vi "OM_ToLabVIEW.vi"(8 "error in (no error)":errorcluster, 10 "DbRow":variant, 11 "Vehicle2 in":refnum<class "Vehicle2.lvclass">) -> (0 "error out":errorcluster, 1 "found":bool, 3 "Vehicle2 out":refnum<class "Vehicle2.lvclass">)   [LabVIEW 2020, in "ORM_Examples.lvlib" / "Vehicle2.lvclass"]
uses:
  Vehicle2.lvclass
  Vehicle2.lvclass/Vehicle2.ctl
  Write Make.vi
  Write Model.vi
  Write Year.vi
  Write VehicleID.vi
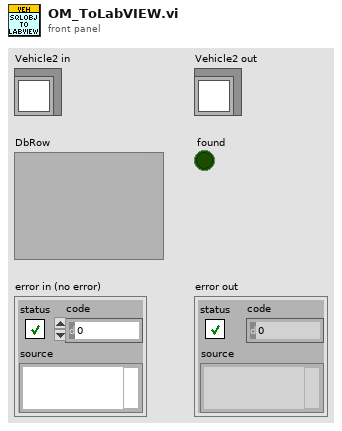
[diagram p1: front panel]
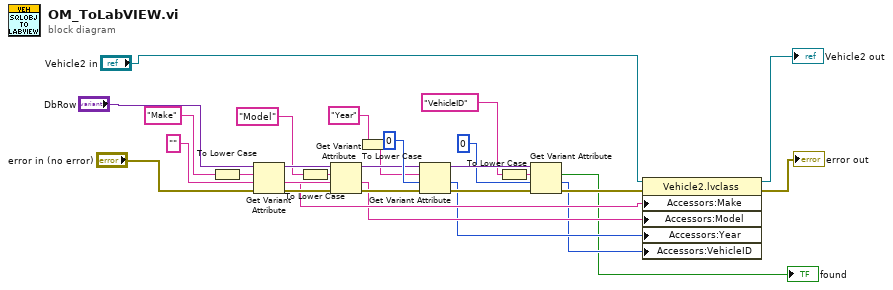
[diagram p0: block diagram]
diagram:
  w22 = "" ("Title")
  n1 = To Lower Case(string="Make" ("Title")) -> (all lower case string=w8:string)
  n2 = Get Variant Attribute(Variant="DbRow", name=w8, default value (empty Variant)=w22, error in="error in (no error)") -> (duplicate Variant=w26:variant, value=w21:string, error out=w24:errorcluster)  [unwired: 1 out]
  n3 = To Lower Case(string="Model" ("Title")) -> (all lower case string=w9:string)
  n4 = Get Variant Attribute(Variant=w26, name=w9, default value (empty Variant)=w22, error in=w24) -> (duplicate Variant=w25:variant, value=w20:string, error out=w23:errorcluster)  [unwired: 1 out]
  n5 = To Lower Case(string="Year" ("Title")) -> (all lower case string=w11:string)
  n6 = Get Variant Attribute(Variant=w25, name=w11, default value (empty Variant)=0 ("Primary Key"), error in=w23) -> (duplicate Variant=w17:variant, value=w19:i32, error out=w28:errorcluster)  [unwired: 1 out]
  n7 = To Lower Case(string="VehicleID" ("Title")) -> (all lower case string=w10:string)
  n8 = Get Variant Attribute(Variant=w17, name=w10, default value (empty Variant)=0, error in=w28) -> (found=→"found":bool, value=w16:i32, error out=w18:errorcluster)  [unwired: 1 out]
  n9 = property class="Vehicle2.lvclass"(reference="Vehicle2 in", error in=w18, "Accessors:Make"=w21, "Accessors:Model"=w20, "Accessors:Year"=w19, "Accessors:VehicleID"=w16) -> (reference out=→"Vehicle2 out":refnum<class "Vehicle2.lvclass">, error out=→"error out":errorcluster)
